vi "FPGA_GetRef.vi"() -> (0 "FPGA_Ref":refnum<k20>)   [LabVIEW 2009]
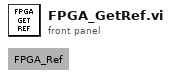
[diagram p1: front panel]
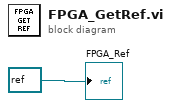
[diagram p0: block diagram]
diagram:
  "FPGA_Ref" <- refnum<k20> refnum ("FPGA VI Reference In")
